vi "SlackAPI-users.conversations.vi"(0 "token":string, 7 "user":string, 11 "error in (no error)":errorcluster) -> (4 "headers":string, 6 "body":string, 15 "error out":errorcluster)   [LabVIEW 2020]
uses:
  <vilib>/httpClient/POSTBuffer.vi
  <vilib>/httpClient/LabVIEWHTTPClient.lvlib
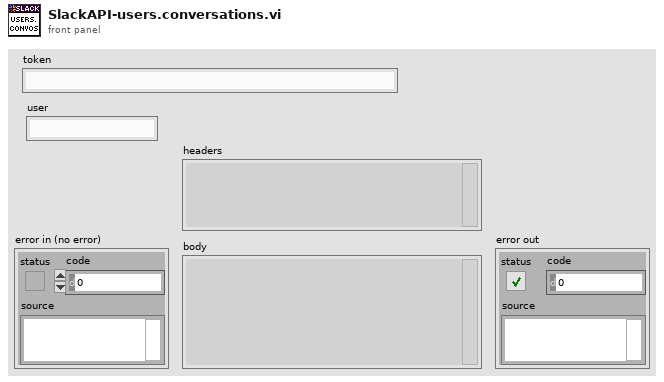
[diagram p1: front panel]
types:
  T1 = typedef "LabVIEWHTTPClient.lvlib/ClientHandle.ctl" = refnum<k1>
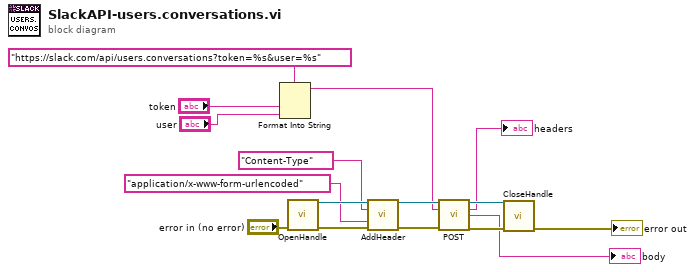
[diagram p0: block diagram]
diagram:
  n1 = Format Into String(format string="https://slack.com/api/users.conversations?token=%s&user=%s", "token", "user") -> (resulting string=w9:string)  [unwired: 2 in, 1 out]
  n2 = call <vilib>:"OpenHandle.vi"("error in (no error)"="error in (no error)") -> ("client handle out"=w15:T1, "error out"=w16:errorcluster)  [unwired: 13 in]
  n3 = call <vilib>:"AddHeader.vi"("client handle"=w15, "header"="Content-Type", "value"="application/x-www-form-urlencoded", "error in (no error)"=w16) -> ("client handle out"=w11:T1, "error out"=w12:errorcluster)  [unwired: 10 in]
  n4 = call-poly <vilib>:"POST.vi"("client handle"=w11, "url"=w9, "error in (no error)"=w12) -> ("client handle out"=w8:T1, "headers"=→"headers":string, "body"=→"body":string, "error out"=w7:errorcluster)  [unwired: 9 in]
  n5 = call <vilib>:"CloseHandle.vi"("client handle"=w8, "error in (no error)"=w7) -> ("error out"=→"error out":errorcluster)  [unwired: 13 in]
